vi "GenerateFilepathLA1.vi"(4 "Auto Date folder":bool, 5 "Filename":string="Spectrometer_", 6 "base path":path=path "M:/Oceanoptics/TDMS test") -> (0 "Numeric":i32, 1 "file path":path=path "M:/Oceanoptics/TDMS test/Spectrometer_test213.tdms", 2 "Folder Path":path)   [LabVIEW 2017]
uses:
  <vilib>/regexp/Match Regular Expression.xnode
panel:
  out "filename":string
  out "Month":string
  out "Year":string
  out "Day":string
  out "date string":string
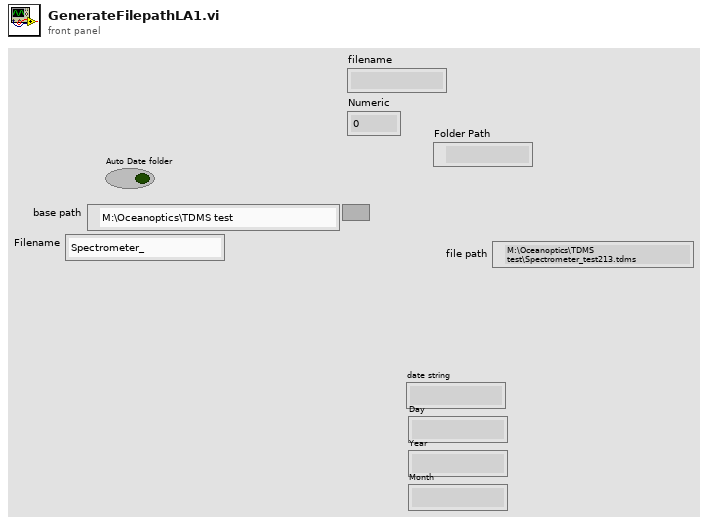
[diagram p1: front panel]
types:
  T1 = enum16{"open", "open or create", "create or replace", "create", "open (read-only)"}
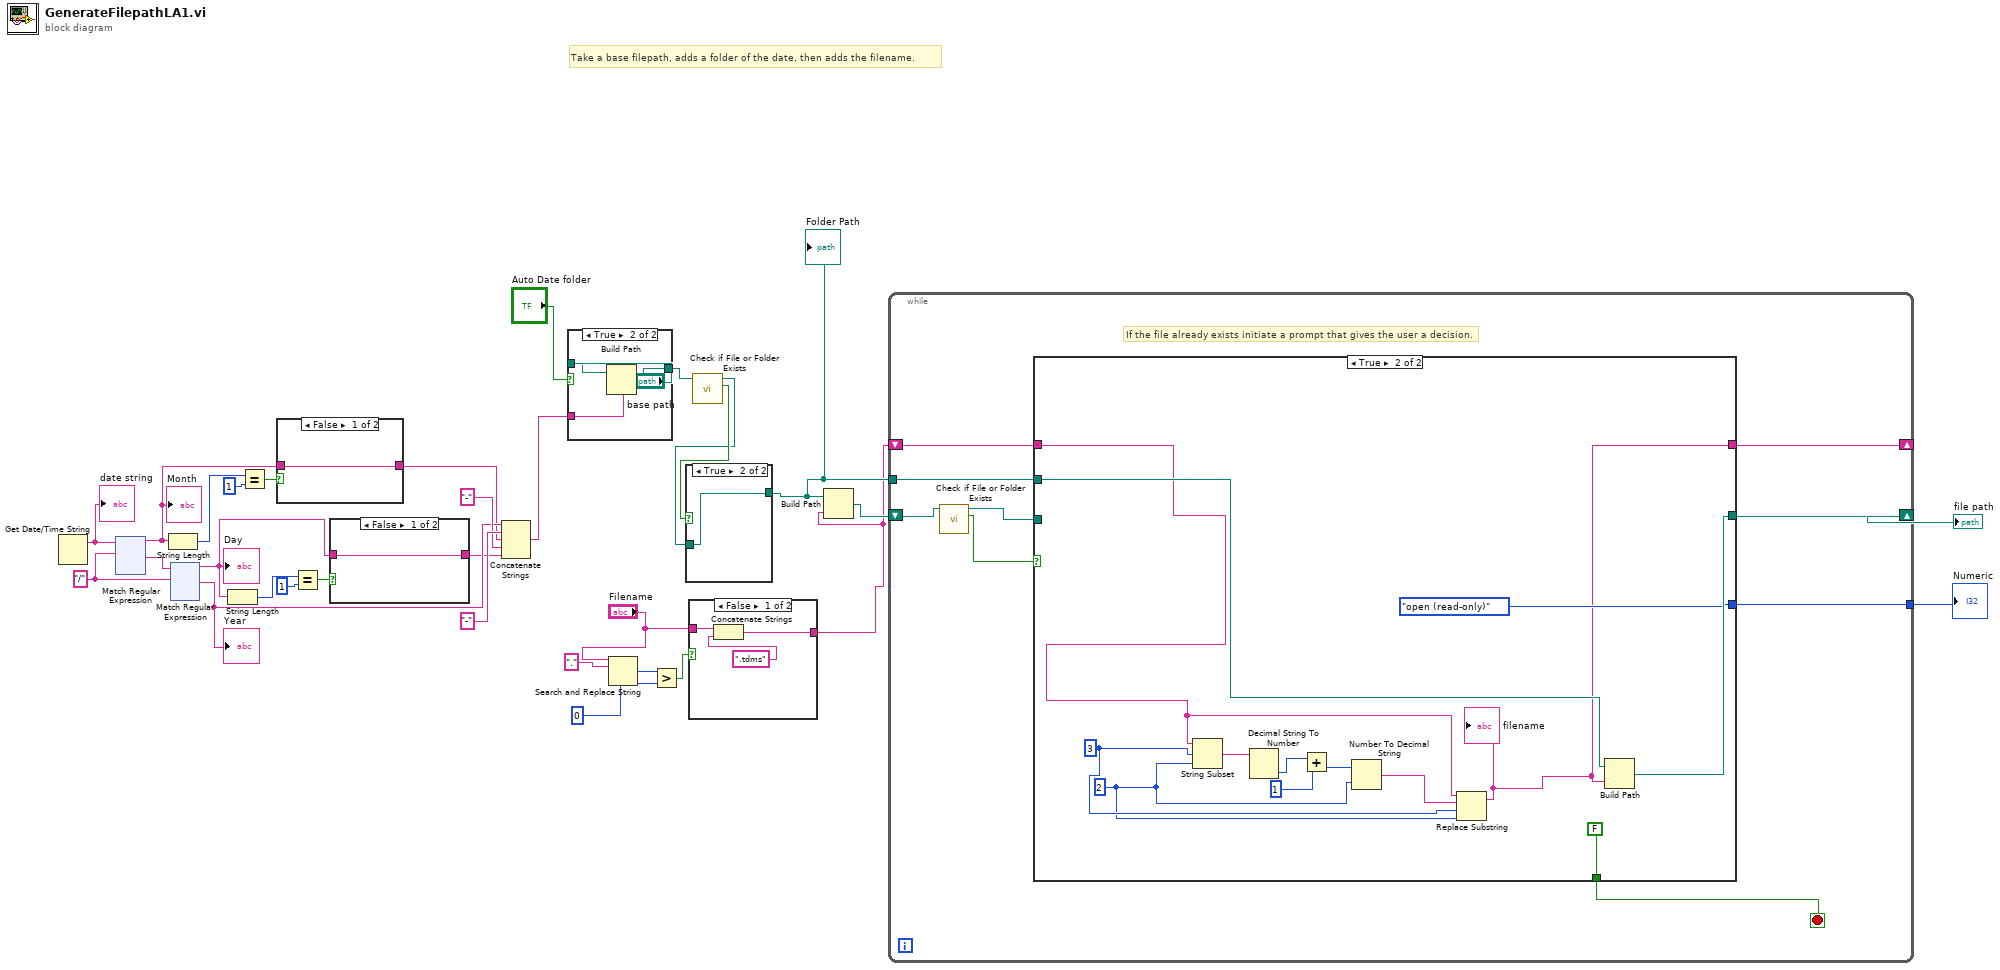
[diagram p0: block diagram]
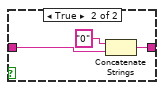
[diagram p3: hidden frame]
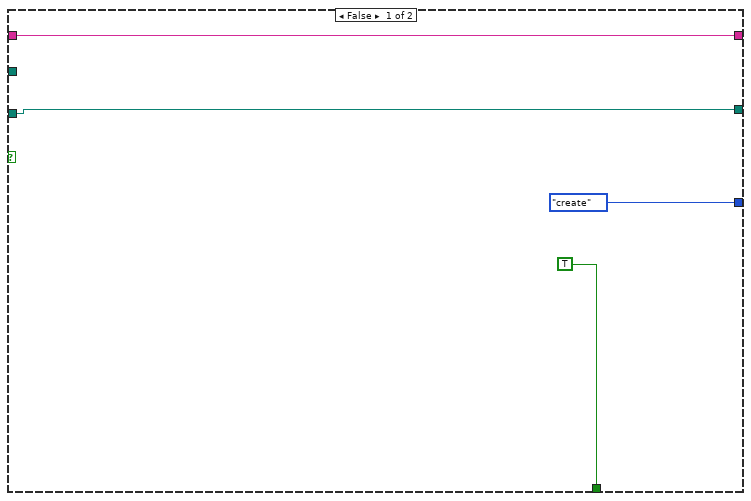
[diagram p4: hidden frame]
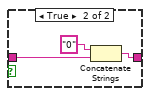
[diagram p5: hidden frame]
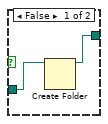
[diagram p6: hidden frame]
diagram:
  w30 = "/" ("regular expression")
  # "Take a base filepath, adds a folder of the date, then adds the filename."
  n1 = Get Date/Time String() -> (date string=w32:string)  [unwired: 3 in, 1 out]
  "date string" <- w32
  n2 = xnode "Match Regular Expression"("input string"=w32, "regular expression"=w30) -> ("before match"=w17:string, "after match"=w31:string)  [unwired: 4 in, 3 out]
  "Month" <- w17
  n3 = String Length(string=w17) -> (length=w20:i32)
  n4 = xnode "Match Regular Expression"("input string"=w31, "regular expression"=w30) -> ("before match"=w9:string, "after match"=w21:string)  [unwired: 4 in, 3 out]
  "Day" <- w9
  "Year" <- w21
  n5 = String Length(string=w9) -> (length=w10:i32)
  n6 = Equal?(x=w20, y=1) -> (x = y?=w18:bool)
  n7 = case shown="False" w18 {
    tunnel: w17 -> [w33 w36]
    tunnel: [w33 w34] -> w16
    frame False {
    }
    frame True {
      n8 = Concatenate Strings("0" ("string"), w36) -> (w34:string)
    }
  }
  n9 = Equal?(x=w10, y=1) -> (x = y?=w12:bool)
  n10 = case shown="False" w12 {
    tunnel: w9 -> [w37 w40]
    tunnel: [w37 w38] -> w8
    frame False {
    }
    frame True {
      n11 = Concatenate Strings("0" ("string"), w40) -> (w38:string)
    }
  }
  n12 = Concatenate Strings(w21, "-" ("string"), w16, "-" ("string"), w8) -> (w25:string)
  n13 = case shown="True" "Auto Date folder" {
    tunnel: "base path" -> [w41 w44]
    tunnel: [w41 w42] -> w24
    tunnel: w25 -> [_ w43]
    frame False {
    }
    frame True {
      n14 = Build Path(base path=w44, name or relative path=w43) -> (appended path=w42:path)
    }
  }
  n15 = Search and Replace String(input string="Filename", search string=".") -> (number of replacements=w4:i32)  [unwired: 6 in, 3 out]
  n16 = Greater?(x=w4, y=0) -> (0:w2:bool)
  n17 = case shown="False" w2 {
    tunnel: [w46 w48] -> w7
    tunnel: "Filename" -> [w45 w48]
    frame False {
      n18 = Concatenate Strings(w45, ".tdms" ("string")) -> (w46:string)
    }
    frame True {
    }
  }
  n19 = call <vilib>:"Check if File or Folder Exists.vi"("path"=w24) -> ("file or folder exists?"=w23:bool, "dup path"=w22:path)  [unwired: 8 in, 1 out]
  n20 = case shown="True" w23 {
    tunnel: w22 -> [w50 w51]
    tunnel: [w49 w51] -> w14
    frame False {
      n21 = Create Folder(path (use dialog)=w50) -> (created path=w49:path)  [unwired: 2 in, 2 out]
    }
    frame True {
    }
  }
  "Folder Path" <- w14
  n22 = Build Path(base path=w14, name or relative path=w7) -> (appended path=w15:path)
  n23 = while {
    tunnel: w14 -> [w55]
    shift-right: [w54] -> w13
    shift-left: w15 -> [w60]
    tunnel: [w53] -> w1
    shift-right: [w52] -> _
    shift-left: w7 -> [w56]
    stop <- w57 stop-if-true
    # "If the file already exists initiate a prompt that gives the user a decision."
    n24 = call <vilib>:"Check if File or Folder Exists.vi"("path"=w60) -> ("file or folder exists?"=w59:bool, "dup path"=w58:path)  [unwired: 8 in, 1 out]
    n25 = case shown="True" w59 {
      tunnel: w58 -> [w63 _]
      tunnel: w56 -> [w61 w70]
      tunnel: [TRUE FALSE] -> w57
      tunnel: w55 -> [_ w72]
      tunnel: [w63 w69] -> w54
      tunnel: [T1."create" ("operation (0:open)") T1."open (read-only)" ("operation (0:open)")] -> w53
      tunnel: [w61 w67] -> w52
      frame False {
      }
      frame True {
        w73 = 3
        w65 = 2
        n26 = String Subset(string=w70, offset (0)=w73, length (rest)=w65) -> (substring=w77:string)
        n27 = Decimal String To Number(string=w77) -> (number=w76:i32)  [unwired: 2 in, 1 out]
        n28 = Add(x=w76, y=1) -> (x+y=w75:i32)
        n29 = Number To Decimal String(number=w75, width (-)=w65) -> (decimal integer string=w74:string)
        n30 = Replace Substring(2:w65, 3:w73, 4:w74, 5:w70) -> (1:w67:string)  [unwired: 1 out]
        "filename" <- w67
        n31 = Build Path(base path=w72, name or relative path=w67) -> (appended path=w69:path)
      }
    }
  }
  "file path" <- w13
  "Numeric" <- w1
